vi "GetSetpoint.vi"(8 "dt":u32, 10 "Start Time":u32, 11 "Profile":cluster{"Pos":dbl, "Vel":dbl, "Accel":dbl}[](array[cluster])) -> (0 "Profile done?":bool, 3 "Setpoints":cluster{"Pos":dbl, "Vel":dbl, "Accel":dbl})   [LabVIEW 2016]
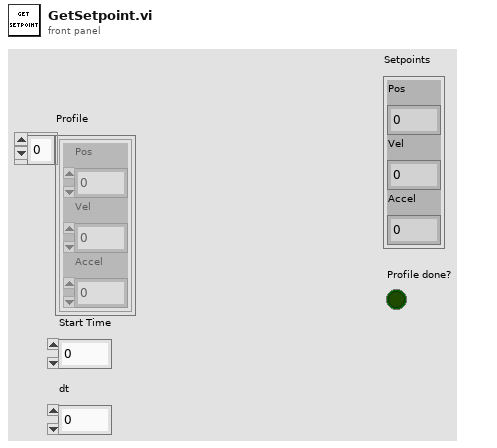
[diagram p1: front panel]
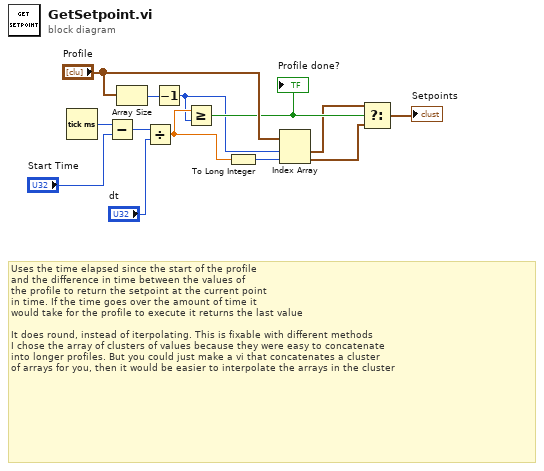
[diagram p0: block diagram]
diagram:
  # "Uses the time elapsed since the start of the profile\nand the difference in time between the values of\nthe profile to return the setpoint at the current point\nin time. If the time goes over the amount of time it\nwould take for the profile to execute it returns the last value\n\nIt does round, instead of iterpolating. This is fixable with different methods\nI chose the array of clusters of values because they were easy to concatenate\ninto longer profiles. But you could just make a vi that concatenates a cluster\nof arrays for you, then it would be easier to interpolate the arrays in the cluster"
  n1 = Tick Count (ms)() -> (millisecond timer value=w13:u32)
  n2 = Subtract(x=w13, y="Start Time") -> (x-y=w11:u32)
  n3 = Array Size(array="Profile") -> (size(s)=w8:i32)
  n4 = Divide(x=w11, y="dt") -> (x/y=w7:dbl)
  n5 = Decrement(x=w8) -> (x-1=w4:i32)
  n6 = Greater Or Equal?(x=w7, y=w4) -> (x >= y?=w6:bool)
  "Profile done?" <- w6
  n7 = To Long Integer(number=w7) -> (32bit integer=w5:i32)
  n8 = Index Array(array="Profile", index #1=w4, index #2=w5) -> (element #1=w3:cluster{"Pos":dbl, "Vel":dbl, "Accel":dbl}, element #2=w2:cluster{"Pos":dbl, "Vel":dbl, "Accel":dbl})
  n9 = Select(t=w3, s=w6, f=w2) -> (s? t:f=→"Setpoints":cluster{"Pos":dbl, "Vel":dbl, "Accel":dbl})
